vi "Resolver Calibration Test Bench.vi"() -> ()   [LabVIEW 2014]
uses:
  <vilib>/Platform/TimedLoop/XDataNode/timing_clust.ctl
  <vilib>/Platform/TimedLoop/XDataNode/nitl_modes.ctl
  <vilib>/Platform/TimedLoop/XDataNode/wakeup.ctl
  CAN/MC/Send Parameter Message.vi
  <vilib>/RioEmbeddedCAN/RioEmbeddedCAN.llb/CANWrite.vi
  <vilib>/Platform/TimedLoop/XDataNode/XDataNode.xnode
  <vilib>/Platform/TimedLoop/XDataNode/XDNodeRunTimeDep.lvlib
panel:
  in  "Spindown":bool
  in  "Requested Torque (Nm)":dbl format="%#_13g"
  in  "CAN Offset":u32=512 format="%x"
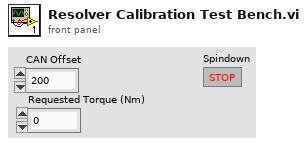
[diagram p1: front panel]
types:
  T1 = typedef "XDNodeRunTimeDep.lvlib/timing_clust.ctl" = cluster{"Expected End [f-1]":u64, "Actual End [f-1]":u64, "Finished Late? [f-1]":bool, "Expected End [i-1]":u64, "Actual End [i-1]":u64, "Finished Late? [i-1]":bool, "Expected Start [i]":u64, "Actual Start [i]":u64, "Expected Start [f]":u64, "Actual Start [f]":u64, "Source Name":string, "Structure Name":string, "Period":i64, "Deadline":i64, "Offset":i64, "Start":i64, "Priority":i32, "Timeout":i32, "Mode":T2, "Wakeup Reason":T3, "Error":errorcluster, "Source Type":string, "Secondary Source Type":string, "Global End Time":u64, "Global Start Time":u64, "Frame Duration":u64, "Iteration Duration":u64, "Assigned CPU":i32, "I/O Scan Engine Mode":u32}
  T2 = typedef "XDNodeRunTimeDep.lvlib/nitl_modes.ctl" = enum32{"No Change", "Process missed periods, maintain original phase", "Discard missed periods, maintain original phase", "Process missed periods, ignore original phase", "Discard missed periods, ignore original phase"}
  T3 = typedef "XDNodeRunTimeDep.lvlib/wakeup.ctl" = enum32{"Normal", "Aborted", "Asynchronous wakeup", "Timing source error", "Timed loop error", "Timeout"}
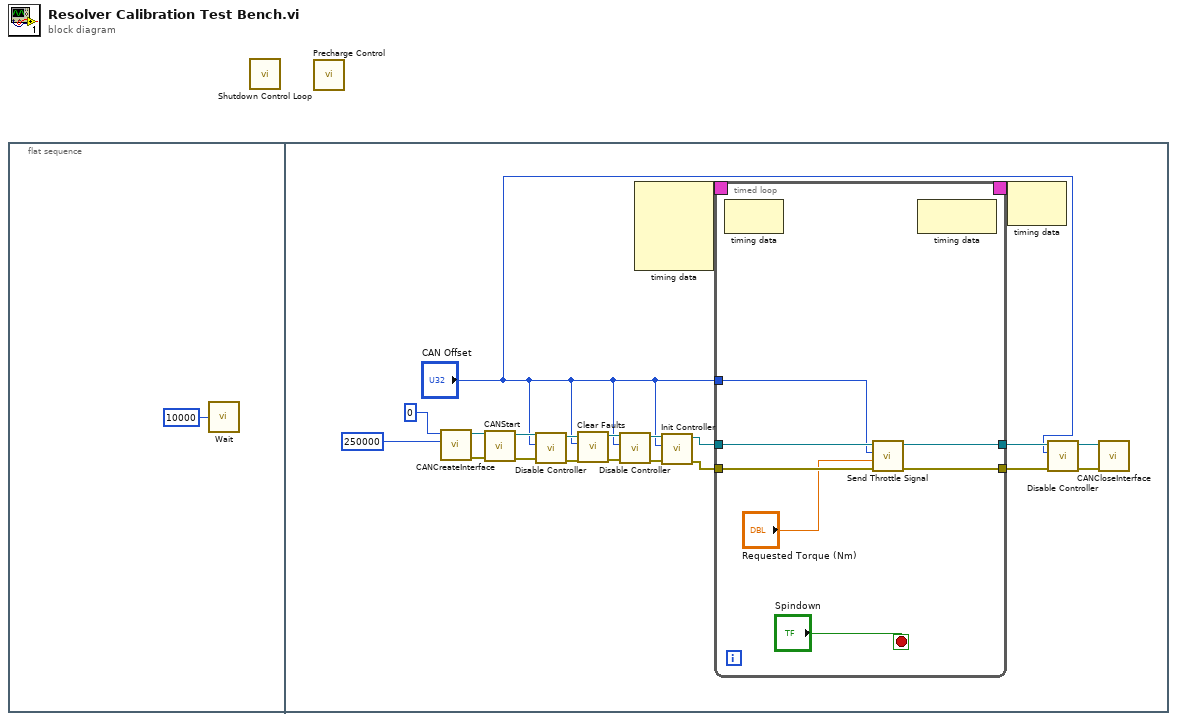
[diagram p0: block diagram]
diagram:
  n1 = flat-sequence {
    frame #0 {
      n2 = call "Wait"("Count(mSec)"=u32 10000) -> ()  [unwired: 1 out]
    }
    frame #1 {
      n3 = call <vilib>:"CANCreateInterface.vi"("baud rate (125000 bps)"=u32 250000, "interface index"=u32 0) -> ("error out"=w18:errorcluster, "interface object out"=w17:refnum<k20>)  [unwired: 8 in]
      n4 = call <vilib>:"CANStart.vi"("error in (no error)"=w18, "interface object in"=w17) -> ("error out"=w15:errorcluster, "interface object out"=w16:refnum<k20>)  [unwired: 8 in]
      n5 = call "Disable Controller.vi"("error in (no error)"=w15, "CAN Offset"="CAN Offset", "interface object in"=w16) -> ("error out"=w3:errorcluster, "interface object out"=w4:refnum<k20>)  [unwired: 7 in]
      n6 = call "Clear Faults.vi"("error in (no error)"=w3, "CAN Offset"="CAN Offset", "interface object in"=w4) -> ("error out"=w5:errorcluster, "interface object out"=w6:refnum<k20>)  [unwired: 7 in]
      n7 = call "Disable Controller.vi"("error in (no error)"=w5, "CAN Offset"="CAN Offset", "interface object in"=w6) -> ("error out"=w7:errorcluster, "interface object out"=w8:refnum<k20>)  [unwired: 7 in]
      n8 = node-c288() -> (w22:T1)  [unwired: 4 in]
      n9 = call "Init Controller.vi"("error in (no error)"=w7, "CAN Offset"="CAN Offset", "interface object in"=w8) -> ("error out"=w13:errorcluster, "interface object out"=w14:refnum<k20>)  [unwired: 7 in]
      n10 = timed-loop {
        timing: w22 -> [_]
        timing-out: [_] -> w21
        tunnel: w14 -> [w29]
        tunnel: w13 -> [w28]
        tunnel: "CAN Offset" -> [w27]
        tunnel: [w24] -> w12
        tunnel: [w23] -> w11
        stop <- "Spindown" stop-if-true
        n11 = node-c288() -> ()  [unwired: 1 in, 1 out]
        n12 = call "Send Throttle Signal.vi"("error in (no error)"=w28, "Requested Torque (Nm)"="Requested Torque (Nm)", "CAN Offset"=w27, "interface object in"=w29) -> ("error out"=w23:errorcluster, "interface object out"=w24:refnum<k20>)  [unwired: 6 in]
        n13 = node-c288() -> ()  [unwired: 1 in, 1 out]
      }
      n14 = node-c288(w21) -> ()  [unwired: 1 out]
      n15 = call "Disable Controller.vi"("error in (no error)"=w11, "CAN Offset"="CAN Offset", "interface object in"=w12) -> ("error out"=w10:errorcluster, "interface object out"=w9:refnum<k20>)  [unwired: 7 in]
      n16 = call <vilib>:"CANCloseInterface.vi"("error in (no error)"=w10, "interface object in"=w9) -> ()  [unwired: 9 in, 1 out]
    }
  }
  n17 = call "Shutdown Control Loop.vi"() -> ()  [unwired: 12 in]
  n18 = call "Precharge Control.vi"() -> ()  [unwired: 12 in]
